vi "Read Command (Hex).vi"(8 "error in (no error)":errorcluster, 11 "Hitronics in":refnum<class "Hitronics.lvclass">) -> (0 "error out":errorcluster, 2 "Command (Hex)":string, 3 "Hitronics out":refnum<class "Hitronics.lvclass">)   [LabVIEW 2018, in "Hitronics.lvlib" / "Hitronics.lvclass"]
uses:
  Hitronics.lvclass
  Hitronics.lvclass/Hitronics.ctl
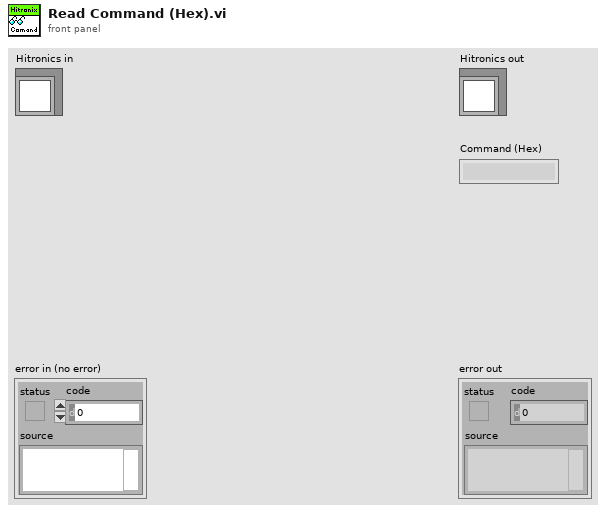
[diagram p1: front panel]
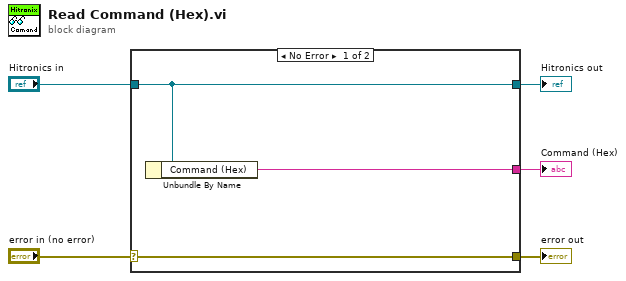
[diagram p0: block diagram]
diagram:
  n1 = case shown="No Error" "error in (no error)" {
    selector: "error in (no error)" -> [w8 w9]
    tunnel: [w8 w9] -> w4
    tunnel: [w7 w10] -> w2
    tunnel: "Hitronics in" -> [w7 w10]
    tunnel: [w6 _] -> w1
    frame No Error {
      n2 = Unbundle By Name(w7) -> ("Command (Hex)"=w6:string)
    }
    frame Error {
    }
  }
  "error out" <- w4
  "Hitronics out" <- w2
  "Command (Hex)" <- w1
